vi "get active element.vi"(8 "error in (no error)":errorcluster) -> (0 "error out":errorcluster, 3 "active_element":string)   [LabVIEW 2019, in "libSimulationControl.lvlib"]
doc: "const char* get_active_element();"
uses:
  libSimulationControl.lvlib
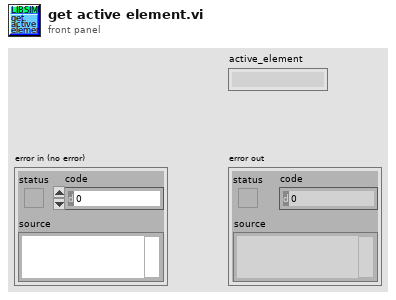
[diagram p1: front panel]
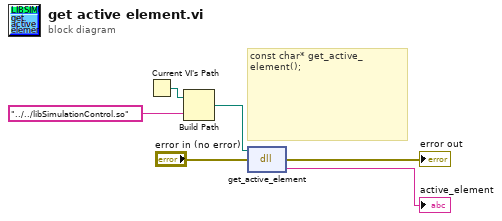
[diagram p0: block diagram]
diagram:
  # "const char* get_active_element();"
  n1 = Current VI's Path() -> (path=w3:path)
  n2 = Build Path(base path=w3, name or relative path="../../libSimulationControl.so") -> (appended path=w1:path)
  n3 = dll-call lib="home/paul/Schreibtisch/Biogas_plant_setup/LabView/lib/libSimulationControl/libSimulationControl.*" fn="get_active_element"(path in=w1, error in="error in (no error)") -> (error out=→"error out":errorcluster, "return type"=→"active_element":string)  [unwired: 1 in, 1 out]
